vi "AddToGroupHelper.vi"(8 "error in (no error)":errorcluster, 9 "Group":string, 10 "Name":string, 11 "Setting Database in":refnum<class "Setting Database.lvclass">) -> (0 "error out":errorcluster, 2 "Active?":bool, 3 "Setting Database out":refnum<class "Setting Database.lvclass">)   [LabVIEW 2019, in "Setting Database.lvclass"]
uses:
  Setting Database.lvclass
  Setting Database.lvclass/Setting Database.ctl
  ObjectSettings/ObjectSettings.lvclass/ObjectSettings.ctl
  ObjectSettings/Accessors/Read Enabled.vi
  ObjectSettings/Accessors/Write Enabled.vi
  Path Settings/Path Settings.lvclass
  C:/Users/Albro/Documents/GitHub/AFM-Lithography/lvsrc/Classes/Settings/ObjectSettings/ObjectSettings.lvclass
  Funnel Settings/Funnel Settings.lvclass
  Dot Settings/Dot Settings.lvclass
  Rectangle Settings/Rectangle Settings.lvclass
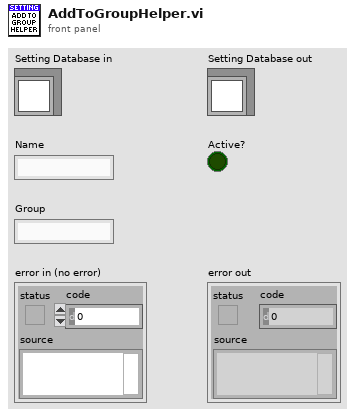
[diagram p1: front panel]
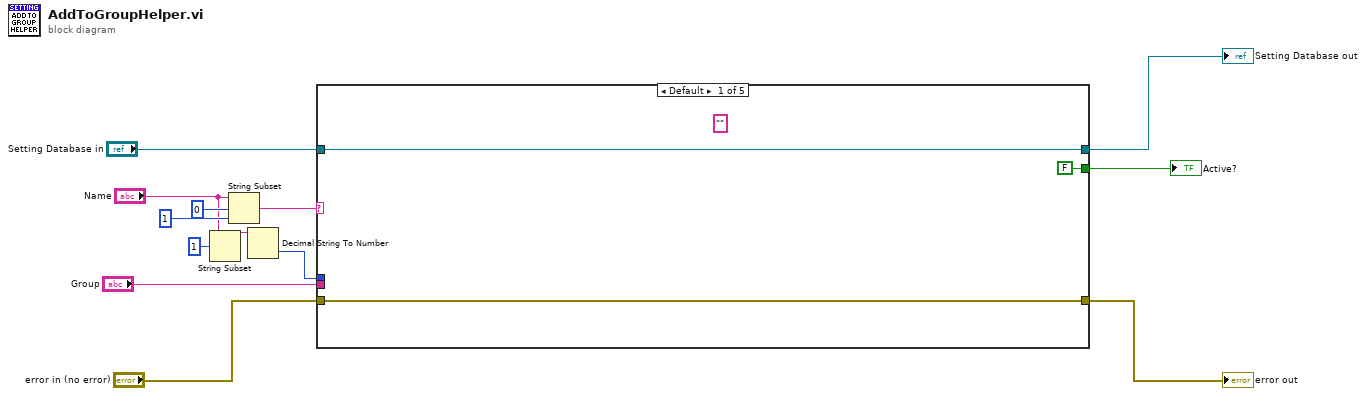
[diagram p0: block diagram]
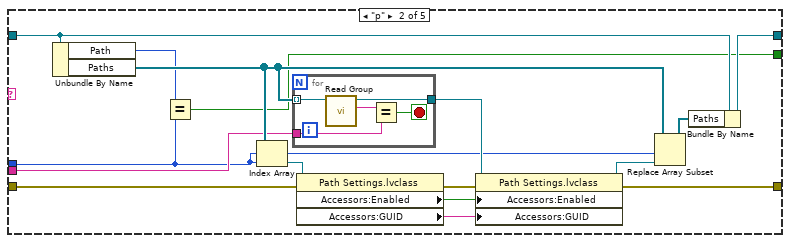
[diagram p2: hidden frame]
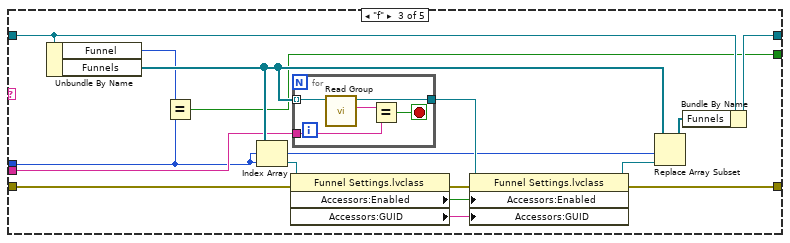
[diagram p3: hidden frame]
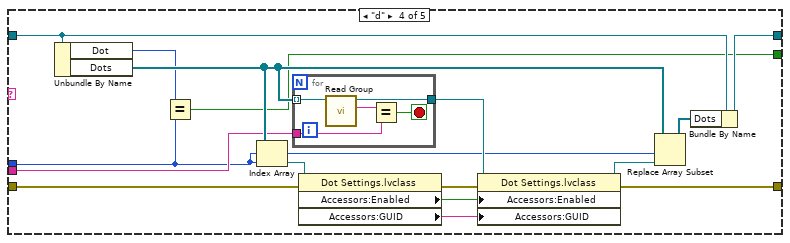
[diagram p4: hidden frame]
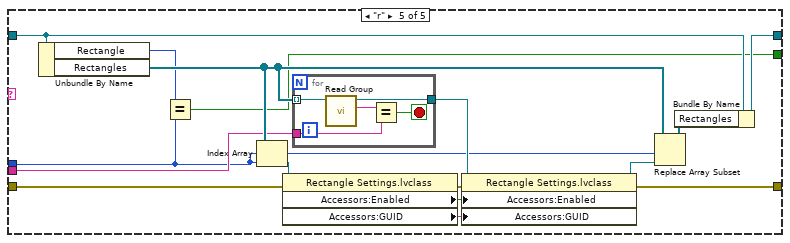
[diagram p5: hidden frame]
diagram:
  n1 = String Subset(string="Name", offset (0)=1) -> (substring=w11:string)  [unwired: 1 in]
  n2 = String Subset(string="Name", offset (0)=0, length (rest)=1 ("length (rest)")) -> (substring=w10:string)
  n3 = Decimal String To Number(string=w11) -> (number=w9:i32)  [unwired: 2 in, 1 out]
  n4 = case shown="Default" w10 {
    tunnel: "Setting Database in" -> [w16 w31 w52 w73 w94]
    tunnel: [w16 w32 w53 w74 w95] -> w7
    tunnel: w9 -> [_ w17 w38 w59 w80]
    tunnel: [w15 w23 w44 w65 w86] -> w5
    tunnel: "error in (no error)" -> [w15 w25 w46 w67 w88]
    tunnel: "Group" -> [_ w28 w49 w70 w91]
    tunnel: [FALSE w19 w40 w61 w82] -> w1
    frame Default {
      (unwired) "" ("States Out")
    }
    frame "p" {
      n5 = Unbundle By Name(w31) -> ("Path"=w18:i32, "Paths"=w29:refnum<class "Path Settings.lvclass">[])
      n6 = Equal?(x=w18, y=w17) -> (x = y?=w19:bool)
      n7 = Index Array(array=w29, index=w17) -> (element=w26:refnum<class "Path Settings.lvclass">)
      n8 = for {
        tunnel: w29 -> [w37] mode=indexing
        tunnel: w28 -> [w35]
        tunnel: [w33] -> w20
        stop <- w34 stop-if-true
        n9 = call-dynamic "Read Group.vi"("ObjectSettings in"=w37) -> ("Group"=w36:string, "ObjectSettings out"=w33:refnum<class "Path Settings.lvclass">)  [unwired: 8 in, 1 out]
        n10 = Equal?(x=w36, y=w35) -> (x = y?=w34:bool)
      }
      n11 = property class="Path Settings.lvclass"(reference=w26, error in=w25) -> (error out=w24:errorcluster, "Accessors:Enabled"=w22:bool, "Accessors:GUID"=w27:string)  [unwired: 1 out]
      n12 = property class="Path Settings.lvclass"(reference=w20, error in=w24, "Accessors:Enabled"=w22, "Accessors:GUID"=w27) -> (reference out=w21:refnum<class "Path Settings.lvclass">, error out=w23:errorcluster)
      n13 = Replace Array Subset(array=w29, new element=w21, index=w17) -> (w30:refnum<class "Path Settings.lvclass">[])
      n14 = Bundle By Name(cluster=w31, "Paths"=w30) -> (w32:refnum<class "Setting Database.lvclass">)
    }
    frame "f" {
      n15 = Unbundle By Name(w52) -> ("Funnel"=w39:i32, "Funnels"=w50:refnum<class "Funnel Settings.lvclass">[])
      n16 = Equal?(x=w39, y=w38) -> (x = y?=w40:bool)
      n17 = Index Array(array=w50, index=w38) -> (element=w47:refnum<class "Funnel Settings.lvclass">)
      n18 = property class="Funnel Settings.lvclass"(reference=w47, error in=w46) -> (error out=w45:errorcluster, "Accessors:Enabled"=w43:bool, "Accessors:GUID"=w48:string)  [unwired: 1 out]
      n19 = for {
        tunnel: w50 -> [w58] mode=indexing
        tunnel: w49 -> [w56]
        tunnel: [w54] -> w41
        stop <- w55 stop-if-true
        n20 = call-dynamic "Read Group.vi"("ObjectSettings in"=w58) -> ("Group"=w57:string, "ObjectSettings out"=w54:refnum<class "Funnel Settings.lvclass">)  [unwired: 8 in, 1 out]
        n21 = Equal?(x=w57, y=w56) -> (x = y?=w55:bool)
      }
      n22 = property class="Funnel Settings.lvclass"(reference=w41, error in=w45, "Accessors:Enabled"=w43, "Accessors:GUID"=w48) -> (reference out=w42:refnum<class "Funnel Settings.lvclass">, error out=w44:errorcluster)
      n23 = Replace Array Subset(array=w50, new element=w42, index=w38) -> (w51:refnum<class "Funnel Settings.lvclass">[])
      n24 = Bundle By Name(cluster=w52, "Funnels"=w51) -> (w53:refnum<class "Setting Database.lvclass">)
    }
    frame "d" {
      n25 = Unbundle By Name(w73) -> ("Dot"=w60:i32, "Dots"=w71:refnum<class "Dot Settings.lvclass">[])
      n26 = Equal?(x=w60, y=w59) -> (x = y?=w61:bool)
      n27 = Index Array(array=w71, index=w59) -> (element=w68:refnum<class "Dot Settings.lvclass">)
      n28 = for {
        tunnel: w71 -> [w79] mode=indexing
        tunnel: w70 -> [w77]
        tunnel: [w75] -> w62
        stop <- w76 stop-if-true
        n29 = call-dynamic "Read Group.vi"("ObjectSettings in"=w79) -> ("Group"=w78:string, "ObjectSettings out"=w75:refnum<class "Dot Settings.lvclass">)  [unwired: 8 in, 1 out]
        n30 = Equal?(x=w78, y=w77) -> (x = y?=w76:bool)
      }
      n31 = property class="Dot Settings.lvclass"(reference=w68, error in=w67) -> (error out=w66:errorcluster, "Accessors:Enabled"=w64:bool, "Accessors:GUID"=w69:string)  [unwired: 1 out]
      n32 = property class="Dot Settings.lvclass"(reference=w62, error in=w66, "Accessors:Enabled"=w64, "Accessors:GUID"=w69) -> (reference out=w63:refnum<class "Dot Settings.lvclass">, error out=w65:errorcluster)
      n33 = Replace Array Subset(array=w71, new element=w63, index=w59) -> (w72:refnum<class "Dot Settings.lvclass">[])
      n34 = Bundle By Name(cluster=w73, "Dots"=w72) -> (w74:refnum<class "Setting Database.lvclass">)
    }
    frame "r" {
      n35 = Unbundle By Name(w94) -> ("Rectangle"=w81:i32, "Rectangles"=w92:refnum<class "Rectangle Settings.lvclass">[])
      n36 = Equal?(x=w81, y=w80) -> (x = y?=w82:bool)
      n37 = Index Array(array=w92, index=w80) -> (element=w89:refnum<class "Rectangle Settings.lvclass">)
      n38 = property class="Rectangle Settings.lvclass"(reference=w89, error in=w88) -> (error out=w87:errorcluster, "Accessors:Enabled"=w85:bool, "Accessors:GUID"=w90:string)  [unwired: 1 out]
      n39 = for {
        tunnel: w92 -> [w100] mode=indexing
        tunnel: w91 -> [w98]
        tunnel: [w96] -> w83
        stop <- w97 stop-if-true
        n40 = call-dynamic "Read Group.vi"("ObjectSettings in"=w100) -> ("Group"=w99:string, "ObjectSettings out"=w96:refnum<class "Rectangle Settings.lvclass">)  [unwired: 8 in, 1 out]
        n41 = Equal?(x=w99, y=w98) -> (x = y?=w97:bool)
      }
      n42 = property class="Rectangle Settings.lvclass"(reference=w83, error in=w87, "Accessors:Enabled"=w85, "Accessors:GUID"=w90) -> (reference out=w84:refnum<class "Rectangle Settings.lvclass">, error out=w86:errorcluster)
      n43 = Replace Array Subset(array=w92, new element=w84, index=w80) -> (w93:refnum<class "Rectangle Settings.lvclass">[])
      n44 = Bundle By Name(cluster=w94, "Rectangles"=w93) -> (w95:refnum<class "Setting Database.lvclass">)
    }
  }
  "error out" <- w5
  "Setting Database out" <- w7
  "Active?" <- w1
